vi "From TCP Connection.vi"(8 "error in (no error)":errorcluster, 10 "Socket":refnum<k5>, 11 "reference in":refnum<class "WebSocket.lvclass">) -> (0 "error out":errorcluster, 1 "FromProcessQueue":refnum<queue>, 2 "ToProcessQueue":refnum<queue>, 3 "reference out":refnum<class "WebSocket.lvclass">)   [LabVIEW 2023, in "WebSocket.lvclass"]
uses:
  WebSocket.lvclass
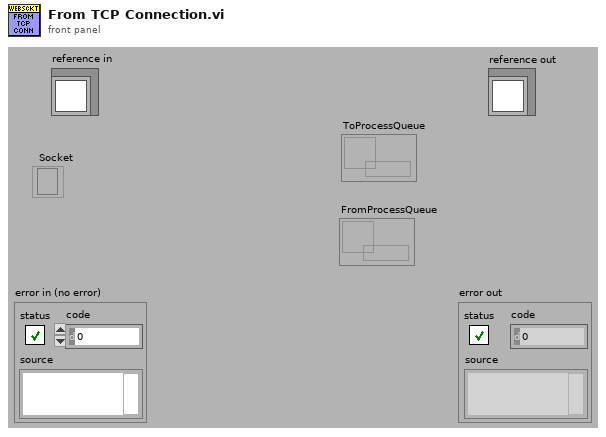
[diagram p1: front panel]
types:
  T1 = typedef "WebSocket.lvclass/ObjectAttributes.ctl" = cluster{"Socket":refnum<k5>, "Thread":refnum<vi>, "From Socket":refnum<queue>, "To Socket":refnum<queue>, "Rx Stats in Progress":variant, "Rx Stats":variant, "Tx Stats in Progress":variant, "Tx Stats":variant}
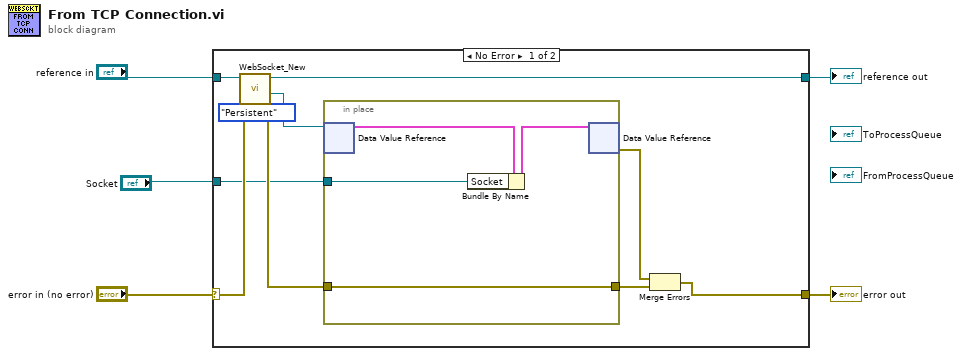
[diagram p0: block diagram]
diagram:
  n1 = case shown="No Error" "error in (no error)" {
    selector: "error in (no error)" -> [w14 w21]
    tunnel: [w7 w21] -> w4
    tunnel: "reference in" -> [w15 w20]
    tunnel: [w6 w20] -> w2
    tunnel: "Socket" -> [w8 _]
    frame No Error {
      n2 = call "WebSocket_New.vi"("Persistent/Debugging(Default)"=enum16{"Default", "Persistent", "NonPersistent"}."Persistent", "error in (no error)"=w14, "reference in"=w15) -> ("error out"=w11:errorcluster, "DVRRefOut"=w12:refnum<data-value>, "reference out"=w6:refnum<class "WebSocket.lvclass">)  [unwired: 5 in, 1 out]
      n3 = in-place {
        in-place-border: w11 -> [w17]
        in-place-border: [w17] -> w10
        in-place-border: w8 -> [w16]
        n4 = in-place-dvr #1(w12) -> (w18:T1)  [unwired: 1 out]
        n5 = Bundle By Name(cluster=w18, "Socket"=w16) -> (w19:T1)
        n6 = in-place-dvr #1(w19) -> (w13:errorcluster)  [unwired: 1 out]
      }
      n7 = Merge Errors(w13, w10) -> (w7:errorcluster)
    }
    frame Error {
    }
  }
  "error out" <- w4
  "reference out" <- w2
